vi "SubVI_Collect_Info.vi"(8 "error in (no error)":errorcluster, 11 "Channel in":T1) -> (0 "error out":errorcluster, 3 "Channel out":T1)   [LabVIEW 2020]
uses:
  <extravilib>/ChannelInstances/Stream-a[.](dbl)/)Channel.ctl
  <extravilib>/ChannelInstances/Stream-a[.](dbl)/EndpointRead.vi
  <extravilib>/ChannelInstances/Stream-a[.](dbl)/Endpoint.vi
  NeuroExo Benchtest Rev1/Global 1.vi
  <extravilib>/ChannelInstances/Stream-a[.](dbl)/)Channel.vi
  <resource>/ChannelSupport/_ChannelSupport/WaitIfNeeded.vi
  <extravilib>/ChannelInstances/Stream-a[.](dbl).lvlib
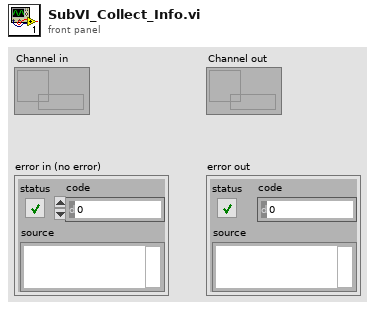
[diagram p1: front panel]
types:
  T1 = typedef "Stream-a[.](dbl).lvlib/)Channel.ctl" = refnum<queue>
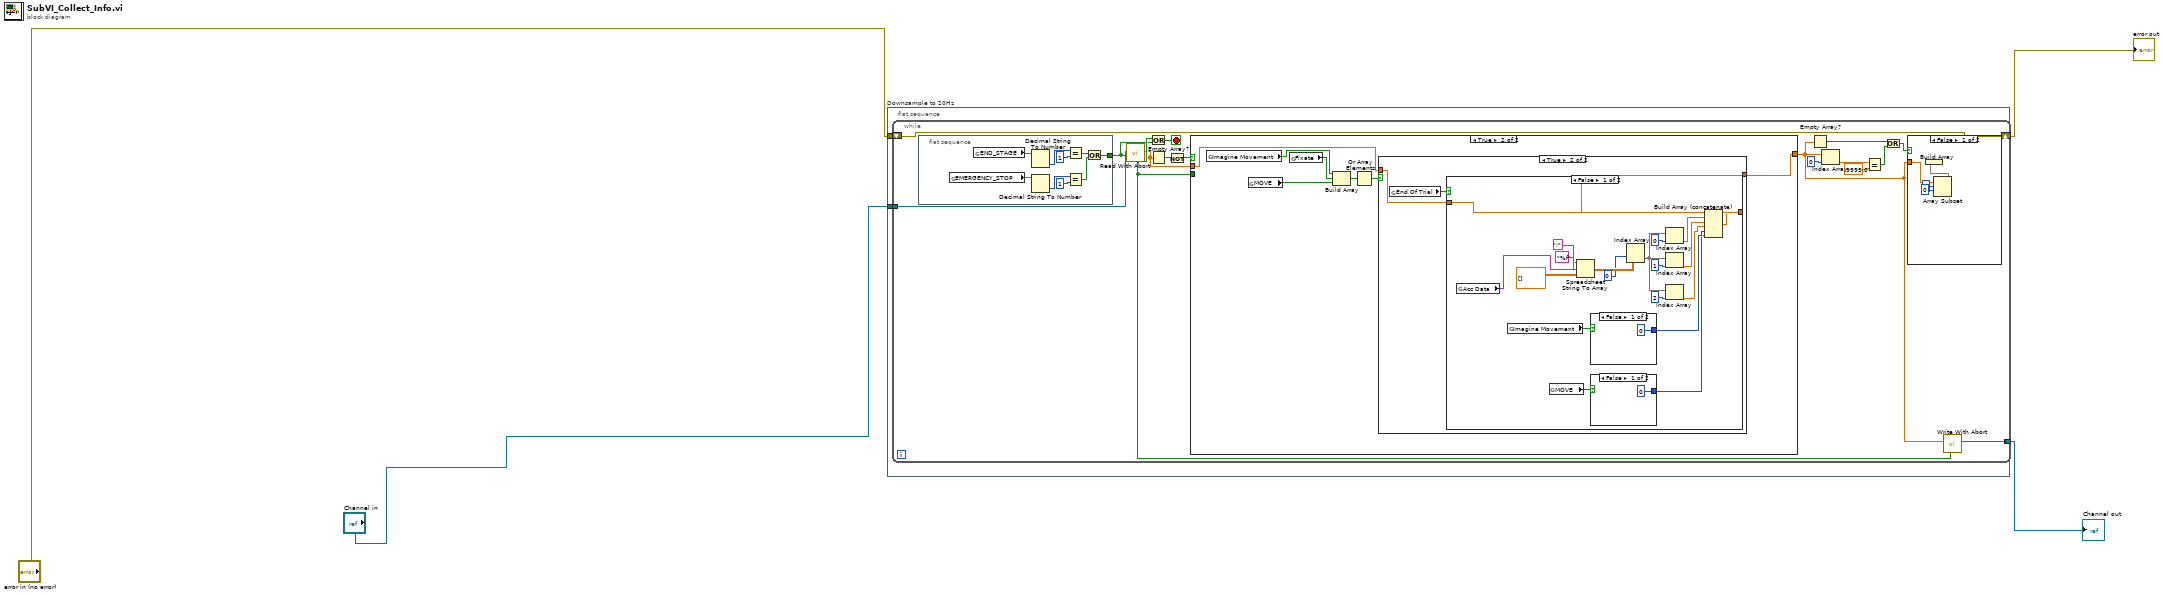
[diagram p0: block diagram]
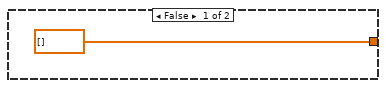
[diagram p3: hidden frame]
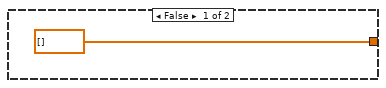
[diagram p4: hidden frame]
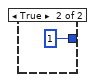
[diagram p5: hidden frame]
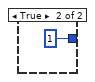
[diagram p6: hidden frame]
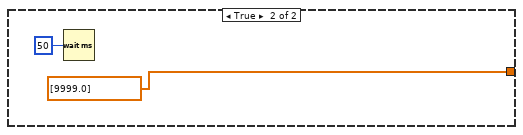
[diagram p7: hidden frame]
diagram:
  n1 = flat-sequence "Downsample to 20Hz" {
    tunnel: [w8] -> w1
    tunnel: [w7] -> w2
    tunnel: "error in (no error)" -> [w6]
    tunnel: "Channel in" -> [w5]
    frame #0 {
      n2 = while {
        tunnel: w5 -> [w24]
        shift-right: [w22] -> w8
        shift-left: w6 -> [w22]
        tunnel: [w20] -> w7
        stop <- w23 stop-if-true
        n3 = flat-sequence {
          tunnel: [w29] -> w19
          frame #0 {
            n4 = global read "Global 1.vi" "EMERGENCY_STOP"() -> (w32:string)
            n5 = global read "Global 1.vi" "END_STAGE"() -> (w37:string)
            n6 = Decimal String To Number(string=w37) -> (number=w36:i32)  [unwired: 2 in, 1 out]
            n7 = Decimal String To Number(string=w32) -> (number=w34:i32)  [unwired: 2 in, 1 out]
            n8 = Equal?(x=w36, y=1) -> (x = y?=w30:bool)
            n9 = Equal?(x=w34, y=1) -> (x = y?=w31:bool)
            n10 = Or(x=w30, y=w31) -> (x .or. y?=w29:bool)
          }
        }
        n11 = call <extravilib>:"Read With Abort.vi"("abort"=w19, "channel"=w24) -> ("element"=w9:dbl[], "aborted?"=w21:bool)  [unwired: 4 in, 4 out]
        n12 = Or(x=w21, y=w19) -> (x .or. y?=w23:bool)
        n13 = Empty Array?(array=w9) -> (empty?=w11:bool)
        n14 = Not(x=w11) -> (.not. x?=w10:bool)
        n15 = case shown="True" w10 {
          tunnel: w9 -> [_ w39]
          tunnel: w21 -> [_ _]
          tunnel: [dbl[] [] w40] -> w12
          frame False {
          }
          frame True {
            n16 = global read "Global 1.vi" "Imagine Movement"() -> (w44:bool)
            n17 = global read "Global 1.vi" "MOVE"() -> (w41:bool)
            n18 = global read "Global 1.vi" "Fixate"() -> (w43:bool)
            n19 = Build Array(w44, w43, w41) -> (w45:bool[])
            n20 = Or Array Elements(Boolean array=w45) -> (logical OR=w42:bool)
            n21 = case shown="True" w42 {
              tunnel: [dbl[] [] w49] -> w40
              tunnel: w39 -> [_ w47]
              frame False {
              }
              frame True {
                n22 = global read "Global 1.vi" "End Of Trial"() -> (w48:bool)
                n23 = case shown="False" w48 {
                  tunnel: [w50 dbl[] [9999.0]] -> w49
                  tunnel: w47 -> [w51 _]
                  frame False {
                    n24 = global read "Global 1.vi" "Acc Data"() -> (w55:string)
                    n25 = global read "Global 1.vi" "Imagine Movement"() -> (w67:bool)
                    n26 = global read "Global 1.vi" "MOVE"() -> (w68:bool)
                    n27 = Spreadsheet String To Array(delimiter (Tab)=";", format string="%f", spreadsheet string=w55, array type (2D Dbl)=dbl[][] []) -> (array=w65:dbl[][])
                    n28 = case shown="False" w67 {
                      tunnel: [0 1] -> w57
                      frame False {
                      }
                      frame True {
                      }
                    }
                    n29 = case shown="False" w68 {
                      tunnel: [0 1] -> w56
                      frame False {
                      }
                      frame True {
                      }
                    }
                    n30 = Index Array(array=w65, index (row)=0 ("disabled index (col)")) -> (element=w64:dbl[])  [unwired: 1 in]
                    n31 = Index Array(array=w64, index=0) -> (element=w52:dbl)
                    n32 = Index Array(array=w64, index=1) -> (element=w53:dbl)
                    n33 = Index Array(array=w64, index=2) -> (element=w54:dbl)
                    n34 = Build Array (concatenate)(w51, w52, w53, w54, w57, w56) -> (w50:dbl[])
                  }
                  frame True {
                    n35 = Wait (ms)(milliseconds to wait=u32 50) -> ()  [unwired: 1 out]
                  }
                }
              }
            }
          }
        }
        n36 = Empty Array?(array=w12) -> (empty?=w14:bool)
        n37 = Index Array(array=w12, index=0) -> (element=w17:dbl)
        n38 = Equal?(x=w17, y=9999.0) -> (x = y?=w15:bool)
        n39 = Or(x=w14, y=w15) -> (x .or. y?=w13:bool)
        n40 = case shown="False" w13 {
          tunnel: w12 -> [w28 _]
          frame False {
            n41 = Array Subset(array=w28, index=0, length=5) -> (w25:dbl[])
            n42 = Build Array(w25) -> ()  [unwired: 1 out]
          }
          frame True {
          }
        }
        n43 = call <extravilib>:"Write With Abort.vi"("abort"=w21, "element"=w12) -> ("channel"=w20:T1)  [unwired: 6 in, 3 out]
      }
    }
  }
  "Channel out" <- w2
  "error out" <- w1
